vi "主界面Z090.vi"() -> ()   [LabVIEW 2013]
uses:
  <vilib>/Utility/error.llb/whitespace.ctl
  <vilib>/Utility/file.llb/Read From Spreadsheet File (string).vi
panel:
  in  "是否取消放行按钮":bool=TRUE
  out "左定长辅具709在位 2":bool
  out "右定长辅具706在位":bool
  out "急停":bool
  out "报警提示":string
  in  "报警号":dbl
  out "本序已做":bool
  out "FGCS":string
  out "KSJJ":string
  out "09rfid":string
  out "上序不合格":bool
  out "上序合格":bool
  out "复位":bool
  in  "右工步号":dbl
  out "右工位操作状态":string
  out "芯片ID":string
  out "本序不合格":bool
  out "权限":string
  out "本序合格":bool
  in  "停止":bool
  in  "左工步号":dbl
  out "产品选型":dbl
  out "左工位操作状态":string
  in  "联线按钮":bool
  in  "选项卡控件":enum32{"自动界面", "手动界面"}(tab)
  out "放回记号笔":bool
  out "取记号笔":bool
  out "放回定长辅具":bool
  out "放回扳手":bool
  out "取扳手":bool
  out "取定长辅具":bool
  out "取螺母":bool
  out "取小卡箍":bool
  out "取大卡箍":bool
  out "毛刷放回":bool
  out "取毛刷":bool
  out "完成，放行按钮":bool
  out "完成，放行按钮":bool
  out "取毛刷":bool
  out "毛刷放回":bool
  out "取大卡箍":bool
  out "取小卡箍":bool
  out "取螺母":bool
  out "取定长辅具":bool
  out "取扳手":bool
  out "放回扳手":bool
  out "放回定长辅具":bool
  out "取记号笔":bool
  out "放回记号笔":bool
  out "左毛刷在位":bool
  out "左定长辅具在位":bool
  out "左扳手在位":bool
  out "左记号笔在位":bool
  out "右毛刷在位":bool
  out "右定长辅具在位":bool
  out "右扳手在位":bool
  out "右记号笔在位":bool
  in  "上阻挡器放行":bool
  in  "下阻挡器放行":bool
  in  "顶升气缸上升":bool
  in  "顶升气缸下降":bool
  out "气缸A上位":bool
  out "上工位检测":bool
  out "通讯状态":bool
  out "急停按钮":bool
  out "气缸A下位":bool
  out "本工位检测":bool
  out "联线状态":bool
  out "光幕保护":bool
  out "气缸B上位":bool
  out "气压报警":bool
  out "下工位检测":bool
  out "RFID触发":bool
  out "气缸B下位":bool
  out "顶升下位":bool
  out "顶升上位":bool
  out "RFID完成":bool
  out "员工ID":string
  out "员工姓名":string
  in  "型号选择":u16(ring)=1 items=["J709", "J706", "J728"]
  in  "参数加载":bool
  out "产品ID":string
  # "芜湖机械转向器装配线"
  # "装护罩，卡箍，外球节"
  # "Q14070机械转向器装配线"
  # "湖北唯思凌科装备制造有限公司 设计开发 (C)2015"
  # "左操作提示"
  # "右操作提示"
  # "辅具在位监测"
  # "辅具在位监测"
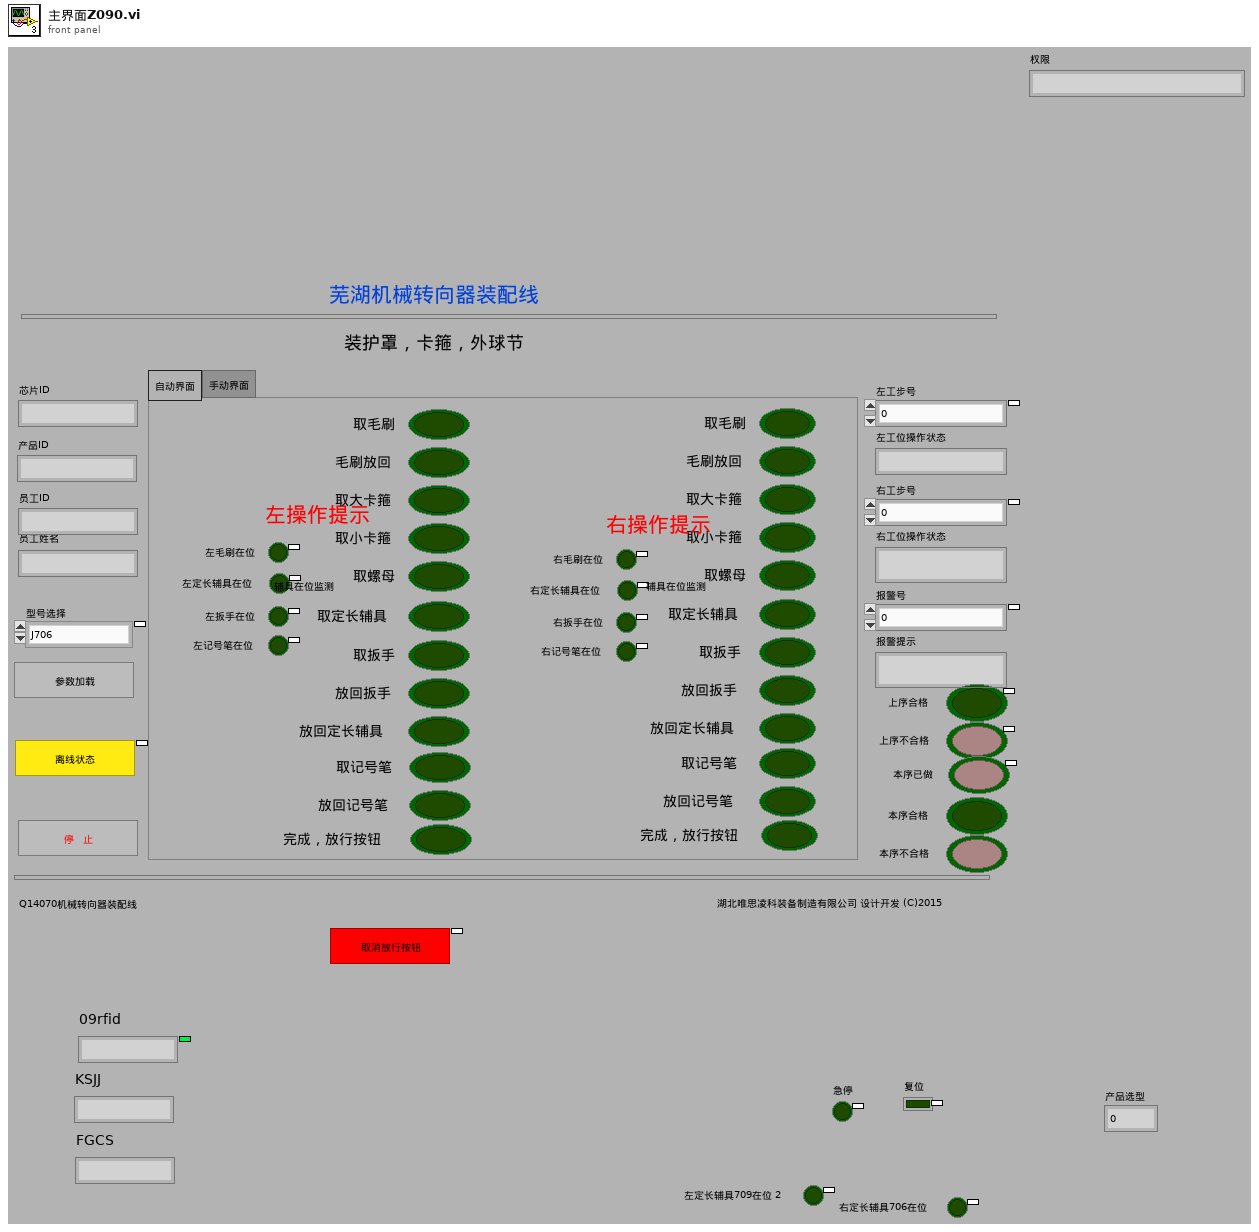
[diagram p1: front panel]
types:
  T1 = typedef "whitespace.ctl" = u16
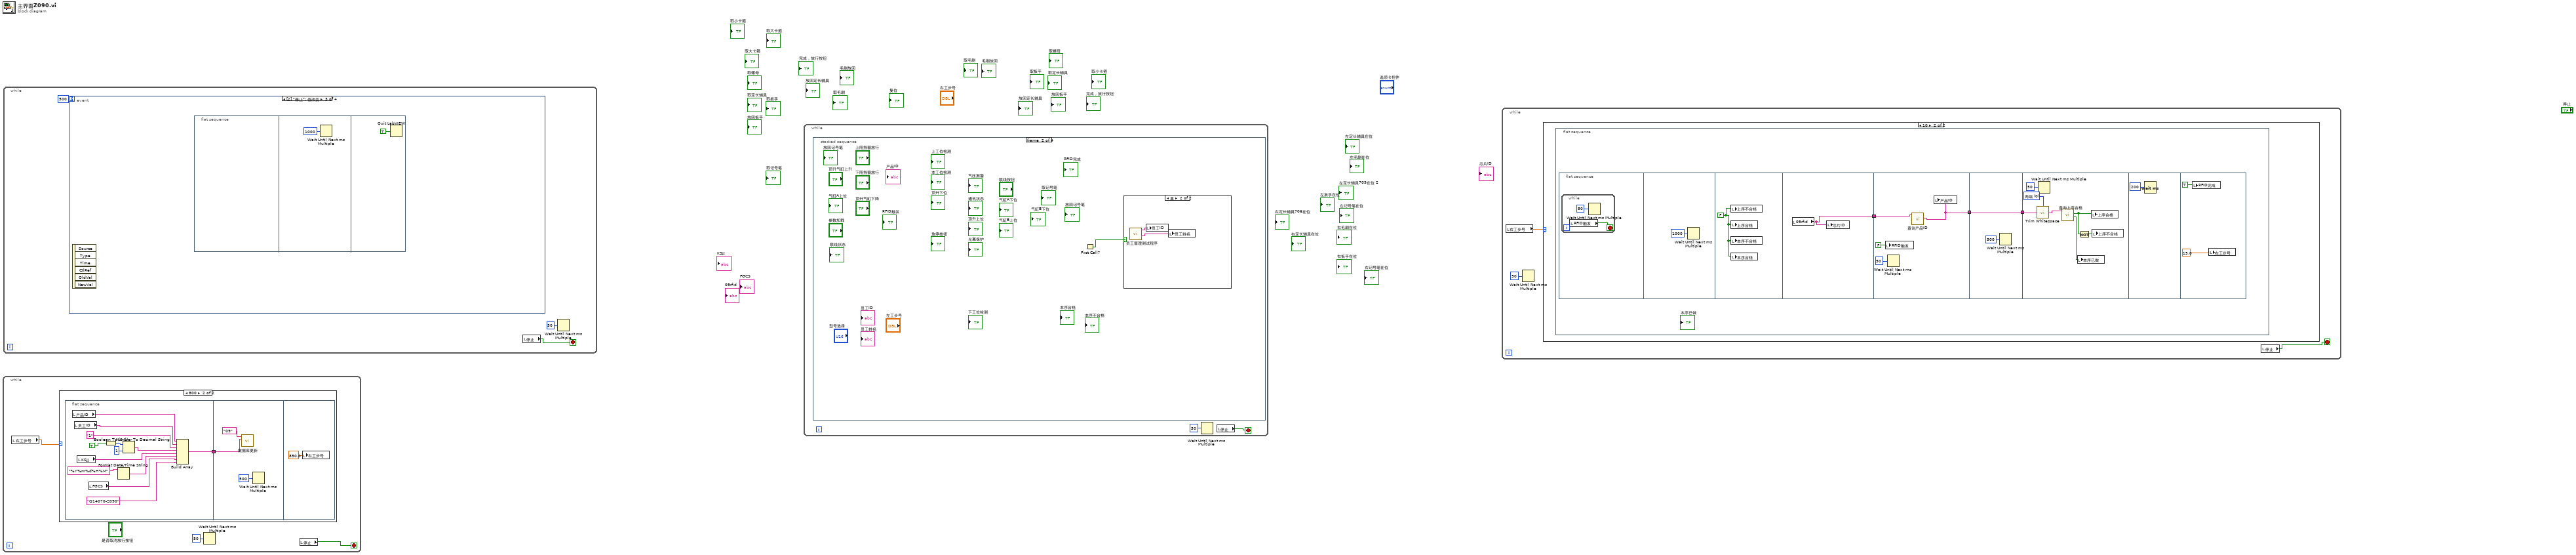
[diagram p0: block diagram]
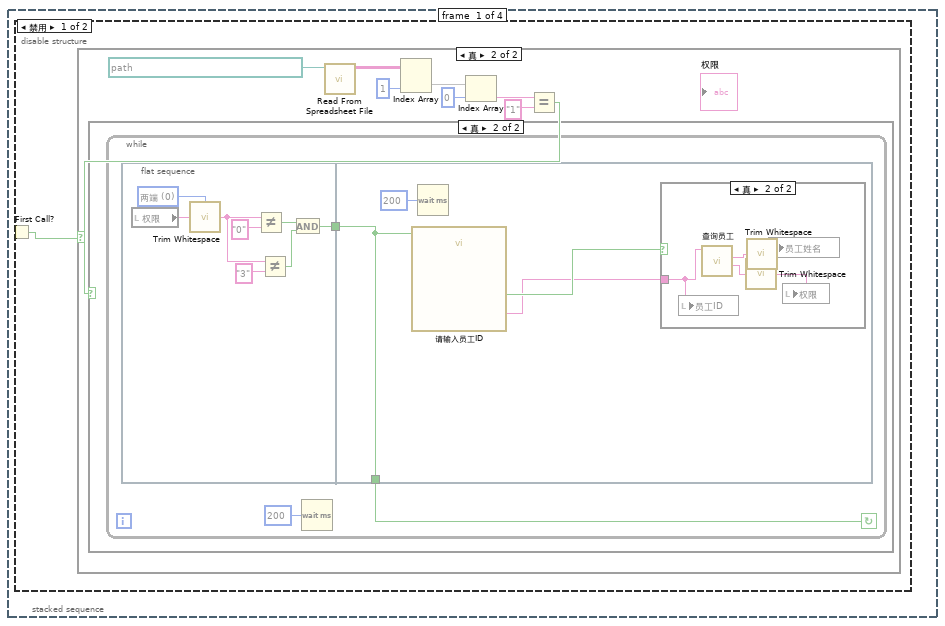
[diagram p4: hidden frame]
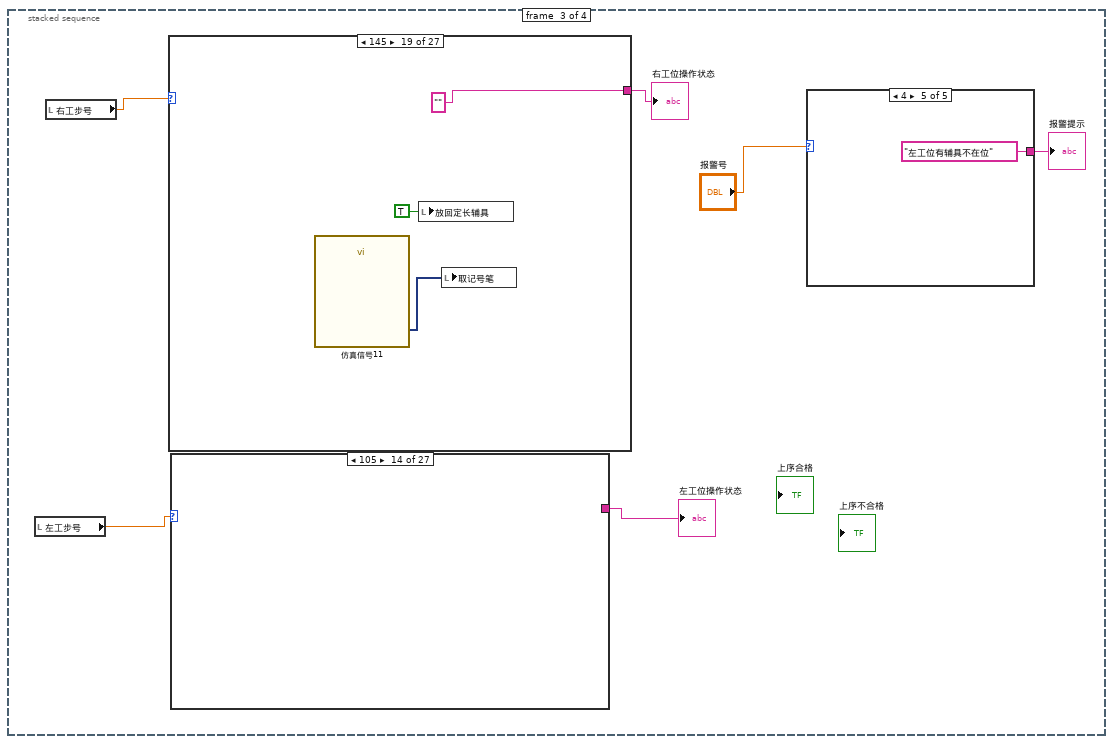
[diagram p10: hidden frame]
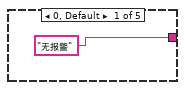
[diagram p11: hidden frame]
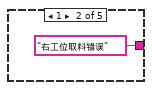
[diagram p12: hidden frame]
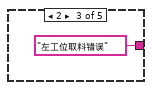
[diagram p13: hidden frame]
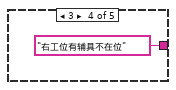
[diagram p14: hidden frame]
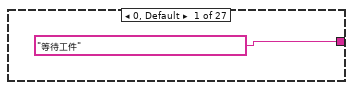
[diagram p15: hidden frame]
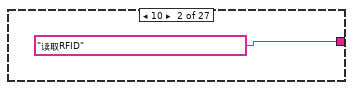
[diagram p16: hidden frame]
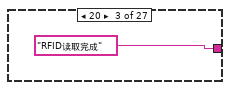
[diagram p17: hidden frame]
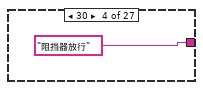
[diagram p18: hidden frame]
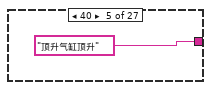
[diagram p19: hidden frame]
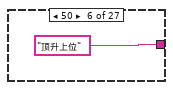
[diagram p20: hidden frame]
diagram:
  n1 = while {
    stop <- w3 stop-if-true
    n2 = local read "右工步号"() -> (w1:dbl)
    n3 = case shown="800" w1 {
      frame 0, Default {
      }
      frame 800 {
        n4 = flat-sequence {
          tunnel: [w7] -> w4
          tunnel: w4 -> [w19]
          frame #0 {
            n5 = local read "产品ID"() -> (w15:string)
            n6 = local read "员工ID"() -> (w5:string)
            n7 = local read "KSJJ"() -> (w12:string)
            n8 = local read "FGCS"() -> (w9:string)
            n9 = Boolean To (0,1)(Boolean=TRUE) -> (0, 1=w17:i16)
            n10 = Format Date/Time String(time format string (%c)="%Y%m%d%H%M" ("时间格式字符串(%c)")) -> (date/time string=w10:string)  [unwired: 2 in]
            n11 = Number To Decimal String(number=w17, width (-)=i16 1 ("宽度(-)")) -> (decimal integer string=w13:string)
            n12 = Build Array(w15, w5, "1", w13, w12, w10, w9, "Q14070-Z090") -> (w7:string[])
          }
          frame #1 {
            n13 = call "数据库更新.vi"("设备号"="09", "数据"=w19) -> ()  [unwired: 13 in, 1 out]
            n14 = Wait Until Next ms Multiple(millisecond multiple=u32 500 ("毫秒倍数")) -> ()  [unwired: 1 out]
          }
          frame #2 {
            n15 = local write "右工步号"(850.0 ("右工步号")) -> ()
          }
        }
      }
    }
    n16 = Wait Until Next ms Multiple(millisecond multiple=u32 50 ("毫秒倍数")) -> ()  [unwired: 1 out]
    n17 = local read "停止"() -> (w3:bool)
  }
  n18 = while {
    stop <- w22 stop-if-true
    n19 = event shown="[2] \"停止\": 值改变" {
      selector: _ -> [_ _ _ _]
      dyn-events: _ -> [_ _ _ _]
      timeout: 500 -> [_ _ _ _]
      event Timeout {
        n20 = event-data() -> ()  [unwired: 3 out]
      }
      event "参数加载": Value Change {
        n21 = event-data() -> ()  [unwired: 7 out]
      }
      event "停止": Value Change {
        n22 = event-data() -> ()  [unwired: 7 out]
        n23 = flat-sequence {
          frame #0 {
          }
          frame #1 {
            n24 = Wait Until Next ms Multiple(millisecond multiple=u32 1000 ("毫秒倍数")) -> ()  [unwired: 1 out]
          }
          frame #2 {
            n25 = Quit LabVIEW(quit? (T)=TRUE ("停止？(T)")) -> ()
          }
        }
      }
      event "产品ID": Value Change {
        n26 = event-data() -> ()  [unwired: 7 out]
        n27 = Format Date/Time String(time format string (%c)="%Y%m%d%H%M" ("时间格式字符串(%c)")) -> (date/time string=w27:string)  [unwired: 2 in]
        n28 = local write "KSJJ"(w27) -> ()
      }
    }
    n29 = local read "停止"() -> (w22:bool)
    n30 = Wait Until Next ms Multiple(millisecond multiple=u32 50 ("毫秒倍数")) -> ()  [unwired: 1 out]
  }
  n31 = while {
    stop <- w29 stop-if-true
    n32 = stacked-sequence {
      frame #0 {
        n33 = disable-structure shown="禁用" {
          frame Disabled {
            n34 = First Call?() -> (First Call?: T/F=w31:bool)
            n35 = case shown="真" w31 {
              frame False {
              }
              frame True {
                n36 = call-poly <vilib>:"Read From Spreadsheet File.vi"("file path (dialog if empty)"=path "\\\\Q113600\\参数/00/管理策略.txt" ("基路径")) -> ("all rows"=w34:string[][])  [unwired: 3 in, 7 out]
                n37 = Index Array(array=w34, index (col)=1 ("索引 (行)")) -> (element=w35:string[])  [unwired: 1 in]
                n38 = Index Array(array=w35, index=0 ("索引")) -> (element=w37:string)
                n39 = Equal?(x=w37, y="1") -> (x = y?=w39:bool)
                n40 = case shown="真" w39 {
                  frame False {
                  }
                  frame True {
                    n41 = while {
                      stop <- w41 continue-if-true
                      n42 = flat-sequence {
                        tunnel: [w47] -> w42
                        tunnel: w42 -> [w51]
                        tunnel: [w51] -> w41
                        frame #0 {
                          w45 = T1 0 items=["两端", "字符串首端", "字符串末端"] ("location (both)")
                          n43 = local read "权限"() -> (w43:string)
                          n44 = call <vilib>:"Trim Whitespace.vi"("string"=w43, "location (both)"=w45) -> ("trimmed string"=w44:string)
                          n45 = Not Equal?(x=w44, y="0") -> (x != y?=w46:bool)
                          n46 = Not Equal?(x=w44, y="3") -> (x != y?=w50:bool)
                          n47 = And(x=w46, y=w50) -> (x .and. y?=w47:bool)
                        }
                        frame #1 {
                          n48 = call "请输入员工ID"("Enable"=w51) -> ("请输入员工ID"=w52:string, "确定"=w53:bool)  [unwired: 1 in, 16 out]
                          n49 = Wait (ms)(milliseconds to wait=u32 200 ("等待时间（毫秒）")) -> ()  [unwired: 1 out]
                          n50 = case shown="真" w53 {
                            tunnel: w52 -> [_ w55]
                            frame False {
                            }
                            frame True {
                              n51 = local write "员工ID"(w55) -> ()
                              n52 = call "查询员工.vi"("员工ID"=w55) -> ("权限"=w58:string, "姓名"=w59:string)  [unwired: 7 in, 2 out]
                              n53 = call <vilib>:"Trim Whitespace.vi"("string"=w58) -> ("trimmed string"=w57:string)  [unwired: 1 in]
                              n54 = call <vilib>:"Trim Whitespace.vi"("string"=w59) -> ("trimmed string"=w56:string)  [unwired: 1 in]
                              n55 = local write "员工姓名"(w56) -> ()
                              n56 = local write "权限"(w57) -> ()
                            }
                          }
                        }
                      }
                      n57 = Wait (ms)(milliseconds to wait=u32 200 ("等待时间（毫秒）")) -> ()  [unwired: 1 out]
                    }
                  }
                }
              }
            }
          }
          frame Enabled {
          }
        }
      }
      frame #1 {
        n58 = First Call?() -> (First Call?: T/F=w60:bool)
        n59 = case shown="真" w60 {
          frame False {
          }
          frame True {
            n60 = call "员工管理测试程序.vi"() -> ("员工姓名"=w62:string, "员工ID"=w61:string)  [unwired: 10 in]
            n61 = local write "员工ID"(w61) -> ()
            n62 = local write "员工姓名"(w62) -> ()
          }
        }
      }
      frame #2 {
        n63 = local read "左工步号"() -> (w66:dbl)
        n64 = local read "右工步号"() -> (w68:dbl)
        n65 = case shown="145" w68 {
          tunnel: ["等待工件" ("工步操作状态") "读取RFID" ("工步操作状态") "RFID读取完成" ("工步操作状态") "阻挡器放行" ("工步操作状态") "顶升气缸顶升" ("工步操作状态") "顶升上位" ("工步操作状态") "取毛刷" ("工步操作状态") "" ("工步操作状态") "" ("工步操作状态") _ "" ("工步操作状态") _ _ _ _ "" ("工步操作状态") "" ("工步操作状态") "" ("工步操作状态") "" ("工步操作状态") _ _ "" ("工步操作状态") "" ("工步操作状态") "" ("工步操作状态") "" ("工步操作状态") "" ("工步操作状态") "" ("工步操作状态")] -> w67
          frame 0, Default {
            w117 = FALSE
            w118 = FALSE
            n66 = local write "完成，放行按钮"(w118) -> ()
            n67 = local write "放回定长辅具"(w118) -> ()
            n68 = local write "放回扳手"(w118) -> ()
            n69 = local write "取扳手"(w118) -> ()
            n70 = local write "取定长辅具"(w118) -> ()
            n71 = local write "毛刷放回"(w118) -> ()
            n72 = local write "取毛刷"(w118) -> ()
            n73 = local write "取小卡箍"(w118) -> ()
            n74 = local write "取大卡箍"(w118) -> ()
            n75 = local write "取螺母"(w118) -> ()
            n76 = local write "放回记号笔"(w118) -> ()
            n77 = local write "取记号笔"(w118) -> ()
            n78 = local write "完成，放行按钮"(w117) -> ()
            n79 = local write "放回扳手"(w117) -> ()
            n80 = local write "取扳手"(w117) -> ()
            n81 = local write "放回定长辅具"(w117) -> ()
            n82 = local write "取定长辅具"(w117) -> ()
            n83 = local write "毛刷放回"(w117) -> ()
            n84 = local write "取毛刷"(w117) -> ()
            n85 = local write "取小卡箍"(w117) -> ()
            n86 = local write "取大卡箍"(w117) -> ()
            n87 = local write "取螺母"(w117) -> ()
            n88 = local write "放回记号笔"(w117) -> ()
            n89 = local write "取记号笔"(w117) -> ()
          }
          frame 10 {
          }
          frame 20 {
          }
          frame 30 {
          }
          frame 40 {
          }
          frame 50 {
          }
          frame 60 {
            n90 = call "仿真信号"() -> ("方波"=w125:dynamicdata)  [unwired: 14 in, 1 out]
            n91 = local write "取毛刷"(w125) -> ()
          }
          frame 70 {
            n92 = call "仿真信号3"() -> ("方波"=w127:dynamicdata)  [unwired: 14 in, 1 out]
            n93 = local write "取毛刷"(TRUE ("取毛刷")) -> ()
            n94 = local write "毛刷放回"(w127) -> ()
          }
          frame 80 {
            n95 = call "仿真信号4"() -> ("方波"=w130:dynamicdata)  [unwired: 14 in, 1 out]
            n96 = local write "毛刷放回"(TRUE ("毛刷放回")) -> ()
            n97 = local write "取大卡箍"(w130) -> ()
          }
          frame 85 {
          }
          frame 90 {
            n98 = call "仿真信号5"() -> ("方波"=w133:dynamicdata)  [unwired: 14 in, 1 out]
            n99 = local write "取大卡箍"(TRUE ("取料监控1")) -> ()
            n100 = local write "取小卡箍"(w133) -> ()
          }
          frame 95 {
          }
          frame 100 {
            n101 = call "仿真信号6"() -> ("方波"=w136:dynamicdata)  [unwired: 14 in, 1 out]
            n102 = local write "取小卡箍"(TRUE ("取料监控2")) -> ()
            n103 = local write "取螺母"(w136) -> ()
          }
          frame 105 {
          }
          frame 110 {
            n104 = call "仿真信号7"() -> ("方波"=w138:dynamicdata)  [unwired: 14 in, 1 out]
            n105 = local write "取螺母"(TRUE ("取料监控3")) -> ()
            n106 = local write "取定长辅具"(w138) -> ()
          }
          frame 120 {
            n107 = call "仿真信号8"() -> ("方波"=w140:dynamicdata)  [unwired: 14 in, 1 out]
            n108 = local write "取定长辅具"(TRUE ("取定长辅具")) -> ()
            n109 = local write "取扳手"(w140) -> ()
          }
          frame 130 {
            n110 = call "仿真信号9"() -> ("方波"=w143:dynamicdata)  [unwired: 14 in, 1 out]
            n111 = local write "取扳手"(TRUE ("取扳手")) -> ()
            n112 = local write "放回扳手"(w143) -> ()
          }
          frame 140 {
            n113 = call "仿真信号10"() -> ("方波"=w146:dynamicdata)  [unwired: 14 in, 1 out]
            n114 = local write "放回扳手"(TRUE ("放回扳手")) -> ()
            n115 = local write "放回定长辅具"(w146) -> ()
          }
          frame 145 {
            n116 = call "仿真信号11"() -> ("方波"=w149:dynamicdata)  [unwired: 14 in, 1 out]
            n117 = local write "放回定长辅具"(TRUE ("放回定长辅具")) -> ()
            n118 = local write "取记号笔"(w149) -> ()
          }
          frame 146 {
            n119 = call "仿真信号12"() -> ("方波"=w152:dynamicdata)  [unwired: 14 in, 1 out]
            n120 = local write "取记号笔"(TRUE ("取记号笔")) -> ()
            n121 = local write "放回记号笔"(w152) -> ()
          }
          frame 147 {
            n122 = call "仿真信号13"() -> ("方波"=w154:dynamicdata)  [unwired: 14 in, 1 out]
            n123 = local write "放回记号笔"(TRUE ("放回记号笔")) -> ()
            n124 = local write "完成，放行按钮"(w154) -> ()
          }
          frame 150 {
            n125 = local write "完成，放行按钮"(TRUE ("完成，放行按钮")) -> ()
          }
          frame 160 {
          }
          frame 170 {
          }
          frame 180 {
          }
          frame 800 {
          }
          frame 900 {
          }
        }
        "右工位操作状态" <- w67
        n126 = case shown="105" w66 {
          tunnel: ["等待工件" ("工步操作状态") "读取RFID" ("工步操作状态") "RFID读取完成" ("工步操作状态") "阻挡器放行" ("工步操作状态") "顶升气缸顶升" ("工步操作状态") "顶升上位" ("工步操作状态") "取毛刷" ("工步操作状态") "" ("工步操作状态") "" ("工步操作状态") _ "" ("工步操作状态") _ _ _ _ "" ("工步操作状态") "" ("工步操作状态") "" ("工步操作状态") _ _ _ "" ("工步操作状态") "" ("工步操作状态") "" ("工步操作状态") "" ("工步操作状态") "" ("工步操作状态") "" ("工步操作状态")] -> w65
          frame 0, Default {
          }
          frame 10 {
          }
          frame 20 {
          }
          frame 30 {
          }
          frame 40 {
          }
          frame 50 {
          }
          frame 60 {
            n127 = call "仿真信号2"() -> ("方波"=w80:dynamicdata)  [unwired: 14 in, 1 out]
            n128 = local write "取毛刷"(w80) -> ()
          }
          frame 70 {
            n129 = call "仿真信号14"() -> ("方波"=w82:dynamicdata)  [unwired: 14 in, 1 out]
            n130 = local write "取毛刷"(TRUE ("取毛刷")) -> ()
            n131 = local write "毛刷放回"(w82) -> ()
          }
          frame 80 {
            n132 = call "仿真信号15"() -> ("方波"=w85:dynamicdata)  [unwired: 14 in, 1 out]
            n133 = local write "毛刷放回"(TRUE ("毛刷放回")) -> ()
            n134 = local write "取大卡箍"(w85) -> ()
          }
          frame 85 {
          }
          frame 90 {
            n135 = call "仿真信号16"() -> ("方波"=w88:dynamicdata)  [unwired: 14 in, 1 out]
            n136 = local write "取大卡箍"(TRUE ("取料监控1")) -> ()
            n137 = local write "取小卡箍"(w88) -> ()
          }
          frame 95 {
          }
          frame 100 {
            n138 = call "仿真信号17"() -> ("方波"=w91:dynamicdata)  [unwired: 14 in, 1 out]
            n139 = local write "取小卡箍"(TRUE ("取料监控2")) -> ()
            n140 = local write "取螺母"(w91) -> ()
          }
          frame 105 {
          }
          frame 110 {
            n141 = call "仿真信号18"() -> ("方波"=w93:dynamicdata)  [unwired: 14 in, 1 out]
            n142 = local write "取螺母"(TRUE ("取料监控3")) -> ()
            n143 = local write "取定长辅具"(w93) -> ()
          }
          frame 120 {
            n144 = call "仿真信号19"() -> ("方波"=w95:dynamicdata)  [unwired: 14 in, 1 out]
            n145 = local write "取定长辅具"(TRUE ("取定长辅具")) -> ()
            n146 = local write "取扳手"(w95) -> ()
          }
          frame 130 {
            n147 = call "仿真信号20"() -> ("方波"=w98:dynamicdata)  [unwired: 14 in, 1 out]
            n148 = local write "取扳手"(TRUE ("取扳手")) -> ()
            n149 = local write "放回扳手"(w98) -> ()
          }
          frame 140 {
            n150 = call "仿真信号21"() -> ("方波"=w101:dynamicdata)  [unwired: 14 in, 1 out]
            n151 = local write "放回扳手"(TRUE ("放回扳手")) -> ()
            n152 = local write "放回定长辅具"(w101) -> ()
          }
          frame 145 {
            n153 = call "仿真信号22"() -> ("方波"=w104:dynamicdata)  [unwired: 14 in, 1 out]
            n154 = local write "放回定长辅具"(TRUE ("放回定长辅具")) -> ()
            n155 = local write "取记号笔"(w104) -> ()
          }
          frame 146 {
            n156 = call "仿真信号23"() -> ("方波"=w106:dynamicdata)  [unwired: 14 in, 1 out]
            n157 = local write "取记号笔"(TRUE ("取记号笔")) -> ()
            n158 = local write "放回记号笔"(w106) -> ()
          }
          frame 147 {
            n159 = call "仿真信号24"() -> ("方波"=w108:dynamicdata)  [unwired: 14 in, 1 out]
            n160 = local write "放回记号笔"(TRUE ("放回记号笔")) -> ()
            n161 = local write "完成，放行按钮"(w108) -> ()
          }
          frame 150 {
            n162 = local write "完成，放行按钮"(TRUE ("放回定长辅具")) -> ()
          }
          frame 160 {
          }
          frame 170 {
          }
          frame 180 {
          }
          frame 800 {
          }
          frame 900 {
          }
        }
        "左工位操作状态" <- w65
        n163 = case shown="4" "报警号" {
          tunnel: ["无报警" ("工步操作状态") "右工位取料错误" ("工步操作状态") "左工位取料错误" ("工步操作状态") "右工位有辅具不在位" ("工步操作状态") "左工位有辅具不在位" ("工步操作状态")] -> w63
          frame 0, Default {
          }
          frame 1 {
          }
          frame 2 {
          }
          frame 3 {
          }
          frame 4 {
          }
        }
        "报警提示" <- w63
      }
      frame #3 {
        n164 = local read "急停"() -> (w164:bool)
        n165 = Not(x=w164) -> (.not. x?=w163:bool)
        n166 = case shown="真" w163 {
          frame False {
          }
          frame True {
            w165 = FALSE
            w166 = FALSE
            n167 = local write "完成，放行按钮"(w166) -> ()
            n168 = local write "放回扳手"(w166) -> ()
            n169 = local write "取扳手"(w166) -> ()
            n170 = local write "放回定长辅具"(w166) -> ()
            n171 = local write "取定长辅具"(w166) -> ()
            n172 = local write "毛刷放回"(w166) -> ()
            n173 = local write "取毛刷"(w166) -> ()
            n174 = local write "取小卡箍"(w166) -> ()
            n175 = local write "取大卡箍"(w166) -> ()
            n176 = local write "取螺母"(w166) -> ()
            n177 = local write "完成，放行按钮"(w165) -> ()
            n178 = local write "放回定长辅具"(w165) -> ()
            n179 = local write "放回扳手"(w165) -> ()
            n180 = local write "取扳手"(w165) -> ()
            n181 = local write "取定长辅具"(w165) -> ()
            n182 = local write "毛刷放回"(w165) -> ()
            n183 = local write "取毛刷"(w165) -> ()
            n184 = local write "取小卡箍"(w165) -> ()
            n185 = local write "取大卡箍"(w165) -> ()
            n186 = local write "取螺母"(w165) -> ()
          }
        }
      }
    }
    n187 = Wait Until Next ms Multiple(millisecond multiple=u32 50 ("毫秒倍数")) -> ()  [unwired: 1 out]
    n188 = local read "停止"() -> (w29:bool)
  }
  n189 = while {
    stop <- w168 stop-if-true
    n190 = local read "右工步号"() -> (w167:dbl)
    n191 = Wait Until Next ms Multiple(millisecond multiple=u32 50 ("毫秒倍数")) -> ()  [unwired: 1 out]
    n192 = case shown="10" w167 {
      frame 0, Default {
      }
      frame 10 {
        n193 = flat-sequence {
          frame #0 {
            n194 = flat-sequence {
              tunnel: [w177] -> w172
              tunnel: [w178] -> w171
              tunnel: w172 -> [w179]
              tunnel: w171 -> [w183]
              tunnel: [w183] -> w170
              tunnel: w170 -> [w189]
              frame #0 {
                n195 = while {
                  stop <- w174 stop-if-true
                  n196 = local read "RFID触发"() -> (w174:bool)
                  n197 = Wait Until Next ms Multiple(millisecond multiple=u32 50 ("毫秒倍数")) -> ()  [unwired: 1 out]
                }
              }
              frame #1 {
                n198 = Wait Until Next ms Multiple(millisecond multiple=u32 1000 ("毫秒倍数")) -> ()  [unwired: 1 out]
              }
              frame #2 {
                w176 = FALSE ("本序合格")
                n199 = local write "上序不合格"(w176) -> ()
                n200 = local write "上序合格"(w176) -> ()
                n201 = local write "本序不合格"(w176) -> ()
                n202 = local write "本序合格"(w176) -> ()
              }
              frame #3 {
                n203 = local read "09rfid"() -> (w177:string)
                n204 = local write "芯片ID"(w177) -> ()
              }
              frame #4 {
                n205 = local write "RFID触发"(FALSE ("RFID读取触发")) -> ()
                n206 = Wait Until Next ms Multiple(millisecond multiple=u32 50 ("毫秒倍数")) -> ()  [unwired: 1 out]
                n207 = call "查询产品ID.vi"("芯片编码"=w179) -> ("产品ID"=w178:string)  [unwired: 8 in, 2 out]
                n208 = local write "产品ID"(w178) -> ()
              }
              frame #5 {
                n209 = Wait Until Next ms Multiple(millisecond multiple=u32 500 ("毫秒倍数")) -> ()  [unwired: 1 out]
              }
              frame #6 {
                w188 = T1 0 items=["两端", "字符串首端", "字符串末端"] ("location (both)")
                n210 = call <vilib>:"Trim Whitespace.vi"("string"=w189, "location (both)"=w188) -> ("trimmed string"=w187:string)
                n211 = Wait Until Next ms Multiple(millisecond multiple=u32 50 ("毫秒倍数")) -> ()  [unwired: 1 out]
                n212 = call "查询上序合格.vi"("产品ID"=w187) -> ("本序已做"=w184:bool, "上序合格"=w186:bool)  [unwired: 8 in, 1 out]
                n213 = local write "本序已做"(w184) -> ()
                n214 = Not(x=w186) -> (.not. x?=w185:bool)
                n215 = local write "上序合格"(w186) -> ()
                n216 = local write "上序不合格"(w185) -> ()
              }
              frame #7 {
                n217 = Wait (ms)(milliseconds to wait=u32 200 ("等待时间（毫秒）")) -> ()  [unwired: 1 out]
              }
              frame #8 {
                n218 = local write "RFID完成"(TRUE ("RFID读取完成")) -> ()
                n219 = local write "右工步号"(15.0 ("工步号")) -> ()
              }
            }
          }
        }
      }
    }
    n220 = local read "停止"() -> (w168:bool)
  }
